vi "save_MPS_SystemRef_hdf.vi"(0 "file path":path, 1 "Device Name":tag="DAQ2", 5 "TxRx_Params":T2={"sample rate"=1000000.0, "Tx freq"=23809.52380952381, "Tx amp"=1.5, "Tx cycles\nSpectroscopy"=500.0, "Bias amp"=2.0, "Bias freq"=11.904761904761905, "Receive range"=5.0, "Bias Periods\nMagnetometry"=5.0, "Tx Freq Division Factor"=42.0, "Drive Periods per Bias"=2000.0, "TX harmonics"=[52631.57894736842, 78947.36842105263, 105263.15789473684, 131578.94736842104, 157894.73684210525, 184210.52631578947, 210526.31578947368, 236842.1052631579]} {"TX harmonics" format="%#_6p"}, 7 "Rx_f0-f8 Units":string, 11 "SRM Stats":T1={"Mean of Mags\nTF Corrected"=[0.11891545467140323, 3.2359956159889795e-06, 4.683456836791031e-06, 2.2974949759077933e-06, 7.335205151756684e-06, 2.2780944083652307e-06, 3.6882771584744806e-06, 3.943947428053956e-06, 5.677081505502577e-06], "Mean of Phase\nTF Corrected"=[1.2189052024941316, 1.3335507267391822, 1.0623290638021972, 1.2312410772168787, -2.3901914592329807, -0.9400489906160769, -0.38268681350318423, -1.5651667523229502, 2.0808572423614278], "Std of Mags\nTF Corrected"=[1.7822550794636106e-06, 1.362064067189915e-06, 1.4384290038051052e-06, 1.2224491171904712e-06, 1.5415851022050893e-06, 1.1506615886407483e-06, 1.5896649122010608e-06, 1.392010277859625e-06, 1.977168509459674e-06], "Std of Phase\nTF Corrected 4"=[0.00044396269347641464, 2.1812626503429993, 0.36980551924146593, 1.6282356086497982, 1.5207696449300456, 1.7213228694360245, 2.6615550793626337, 0.5214361017901513, 1.6763493877670135], "All Mag"=[], "All Phase"=[], "RxFFTMag_AllFreqs"=[], "RxFFTPhase_AllFreqs"=[], "Std-RxFFT_AllFreqs"=[], "Rx_PSD_AllFreqs"=[], "Std-Rx_PSD_AllFreqs"=[], "TxFFTMag_AllFreqs"=[], "TxFFTPhase_AllFreqs"=[], "Std-TxFFT_AllFreqs"=[], "freqs"=[]}, 12 "Study and Experiment Description":T4={"Study Number"=5, "Study Name"="", "UUID"="", "GUI Open Time"="", "Notes"=""}, 14 "Scanner Description":T3={"Scanner Name"="", "Hardware description"="", "Preamplifier Used"="", "Preamp Gain"=5.0, "Drive Amplifier"="", "Bias Amplifier"="", "Drive Current Monitor"="", "Bias Current Monitor"=""}, 15 "Points from home to max":i32) -> ()   [LabVIEW 2021]
uses:
  <vilib>/UPVI/lvhdf5/file.llb/LVH5F Operation.ctl
  <vilib>/Utility/miscctls.llb/LVRectTypeDef.ctl
  <vilib>/UPVI/lvhdf5/attribute.llb/LVH5A Operation.ctl
  <vilib>/UPVI/lvhdf5/group.llb/H5G_obj_t.ctl
  <vilib>/UPVI/lvhdf5/dataset.llb/LVH5D Operation.ctl
  <vilib>/UPVI/lvhdf5/identifier.llb/Not an HDF5 Refnum Constant.vi
  <vilib>/UPVI/lvhdf5/attribute.llb/Write Multiple Attributes.vi
  MPS_global_variables.vi
  <vilib>/UPVI/lvhdf5/utility.llb/Select HDF5 Dialog.vi
  <vilib>/UPVI/lvhdf5/utility.llb/Select HDF5 Dialog (Object Only).vi
  <vilib>/UPVI/lvhdf5/dataset.llb/Simple H5Dwrite (Variant).vi
  <vilib>/UPVI/lvhdf5/common.llb/To HDF5 Ref.vi
  <vilib>/UPVI/lvhdf5/dataset.llb/H5Dclose.vi
  <vilib>/UPVI/lvhdf5/attribute.llb/LVH5 Write Attributes.xnode
  <vilib>/UPVI/lvhdf5/library.llb/HDF5 Ref.ctl
  <vilib>/UPVI/lvhdf5/dataset.llb/Write Dataset with Attributes.xnode
  <vilib>/UPVI/lvhdf5/attribute.llb/Cluster to Attribute Array.xnode
  <vilib>/Utility/error.llb/Error Cluster From Error Code.vi
  <vilib>/UPVI/lvhdf5/dataset.llb/OpenCreateReplace Dataset by Element Type.vi
  <vilib>/UPVI/lvhdf5/dataspace.llb/H5Sselect_hyperslab.vi
  <vilib>/UPVI/lvhdf5/dataset.llb/H5Dwrite (Variant).vi
  <vilib>/UPVI/lvhdf5/dataset.llb/H5Dget_space.vi
  <vilib>/UPVI/lvhdf5/attribute.llb/private/LVH5AwriteWDTAttrs.vi
  <vilib>/UPVI/lvhdf5/dataspace.llb/H5Sclose.vi
  <vilib>/UPVI/lvhdf5/utility.llb/Select HDF5 Dialog (File and Object).vi
  <resource>/objmgr/daqmx.rc
  <vilib>/UPVI/lvhdf5/library.llb/HDF5 Ref.lvclass
  <vilib>/Utility/Data Type/Get Type Information.vi
  <vilib>/Utility/Data Type/NI_Data Type.lvlib
  <vilib>/Utility/Data Type/Get Cluster Information.vi
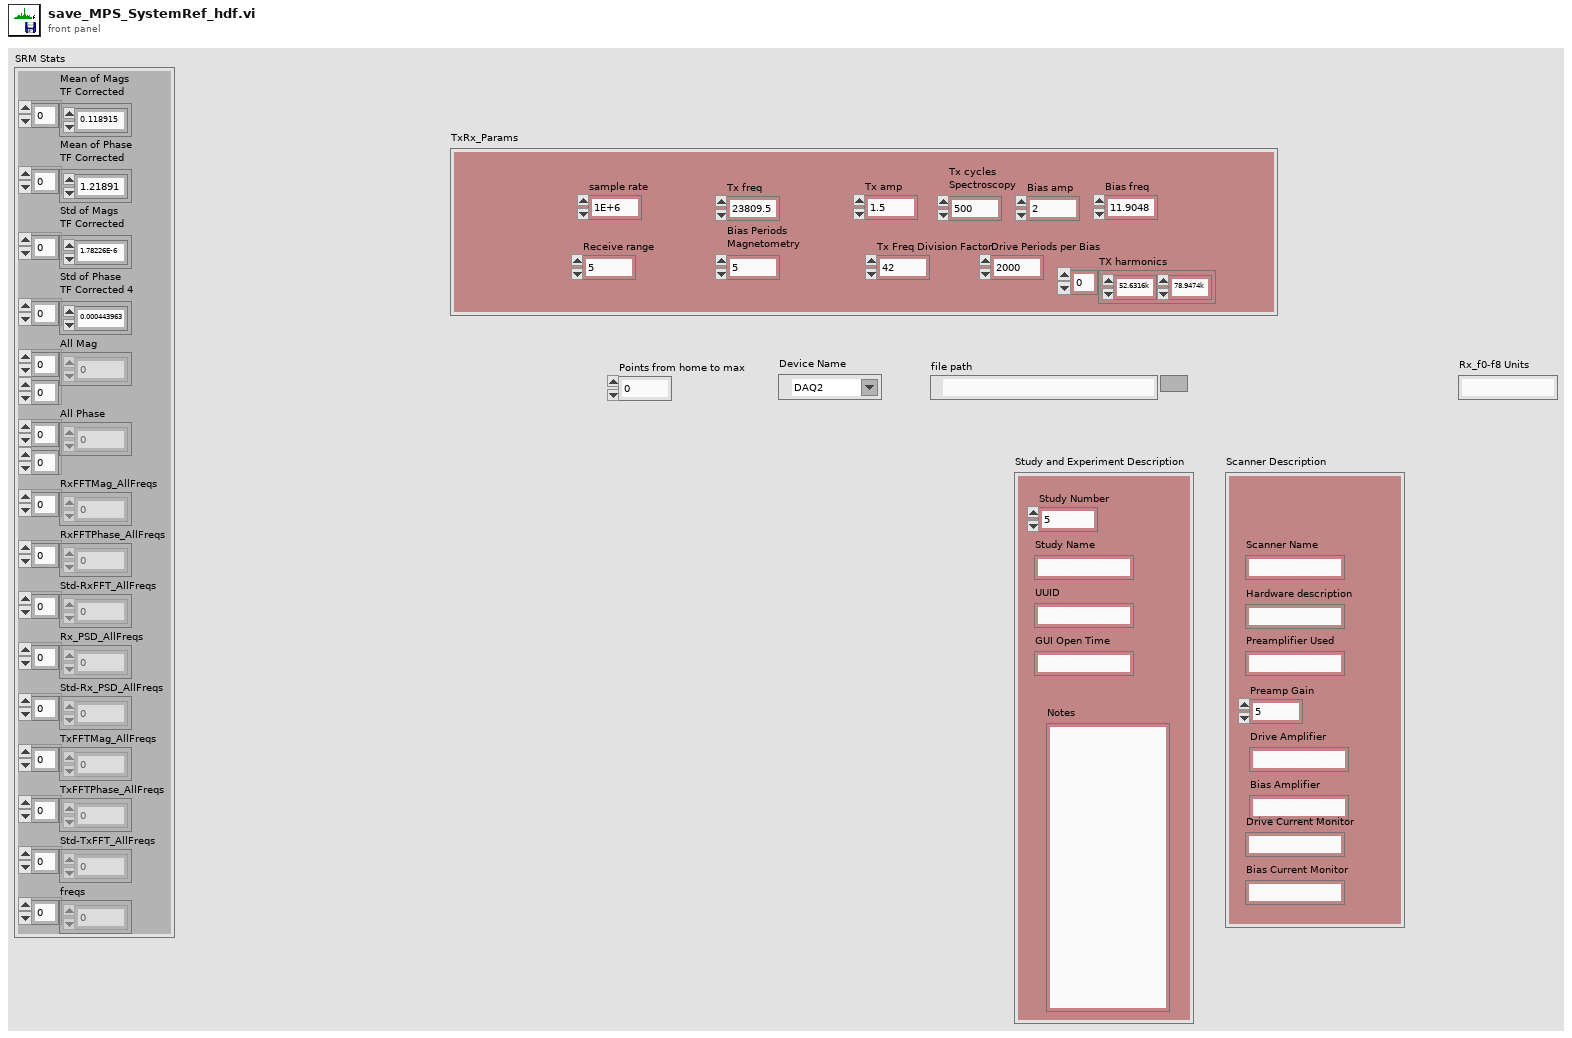
[diagram p1: front panel]
types:
  T1 = cluster{"Mean of Mags\nTF Corrected":dbl[], "Mean of Phase\nTF Corrected":dbl[], "Std of Mags\nTF Corrected":dbl[], "Std of Phase\nTF Corrected 4":dbl[], "All Mag":dbl[][], "All Phase":dbl[][], "RxFFTMag_AllFreqs":dbl[], "RxFFTPhase_AllFreqs":dbl[], "Std-RxFFT_AllFreqs":dbl[], "Rx_PSD_AllFreqs":dbl[], "Std-Rx_PSD_AllFreqs":dbl[], "TxFFTMag_AllFreqs":dbl[], "TxFFTPhase_AllFreqs":dbl[], "Std-TxFFT_AllFreqs":dbl[], "freqs":dbl[]}
  T2 = cluster{"sample rate":dbl, "Tx freq":dbl, "Tx amp":dbl, "Tx cycles\nSpectroscopy":dbl, "Bias amp":dbl, "Bias freq":dbl, "Receive range":dbl, "Bias Periods\nMagnetometry":dbl, "Tx Freq Division Factor":dbl, "Drive Periods per Bias":dbl, "TX harmonics":dbl[]}
  T3 = cluster{"Scanner Name":string, "Hardware description":string, "Preamplifier Used":string, "Preamp Gain":dbl, "Drive Amplifier":string, "Bias Amplifier":string, "Drive Current Monitor":string, "Bias Current Monitor":string}
  T4 = cluster{"Study Number":i64, "Study Name":string, "UUID":string, "GUI Open Time":string, "Notes":string}
  T5 = typedef "LVH5F Operation.ctl" = enum16{"open", "open or create", "create or replace", "create or replace (with confirmation)", "create", "open (read only)"}
  T6 = typedef "HDF5 Ref.ctl" = refnum<class "HDF5 Ref.lvclass">
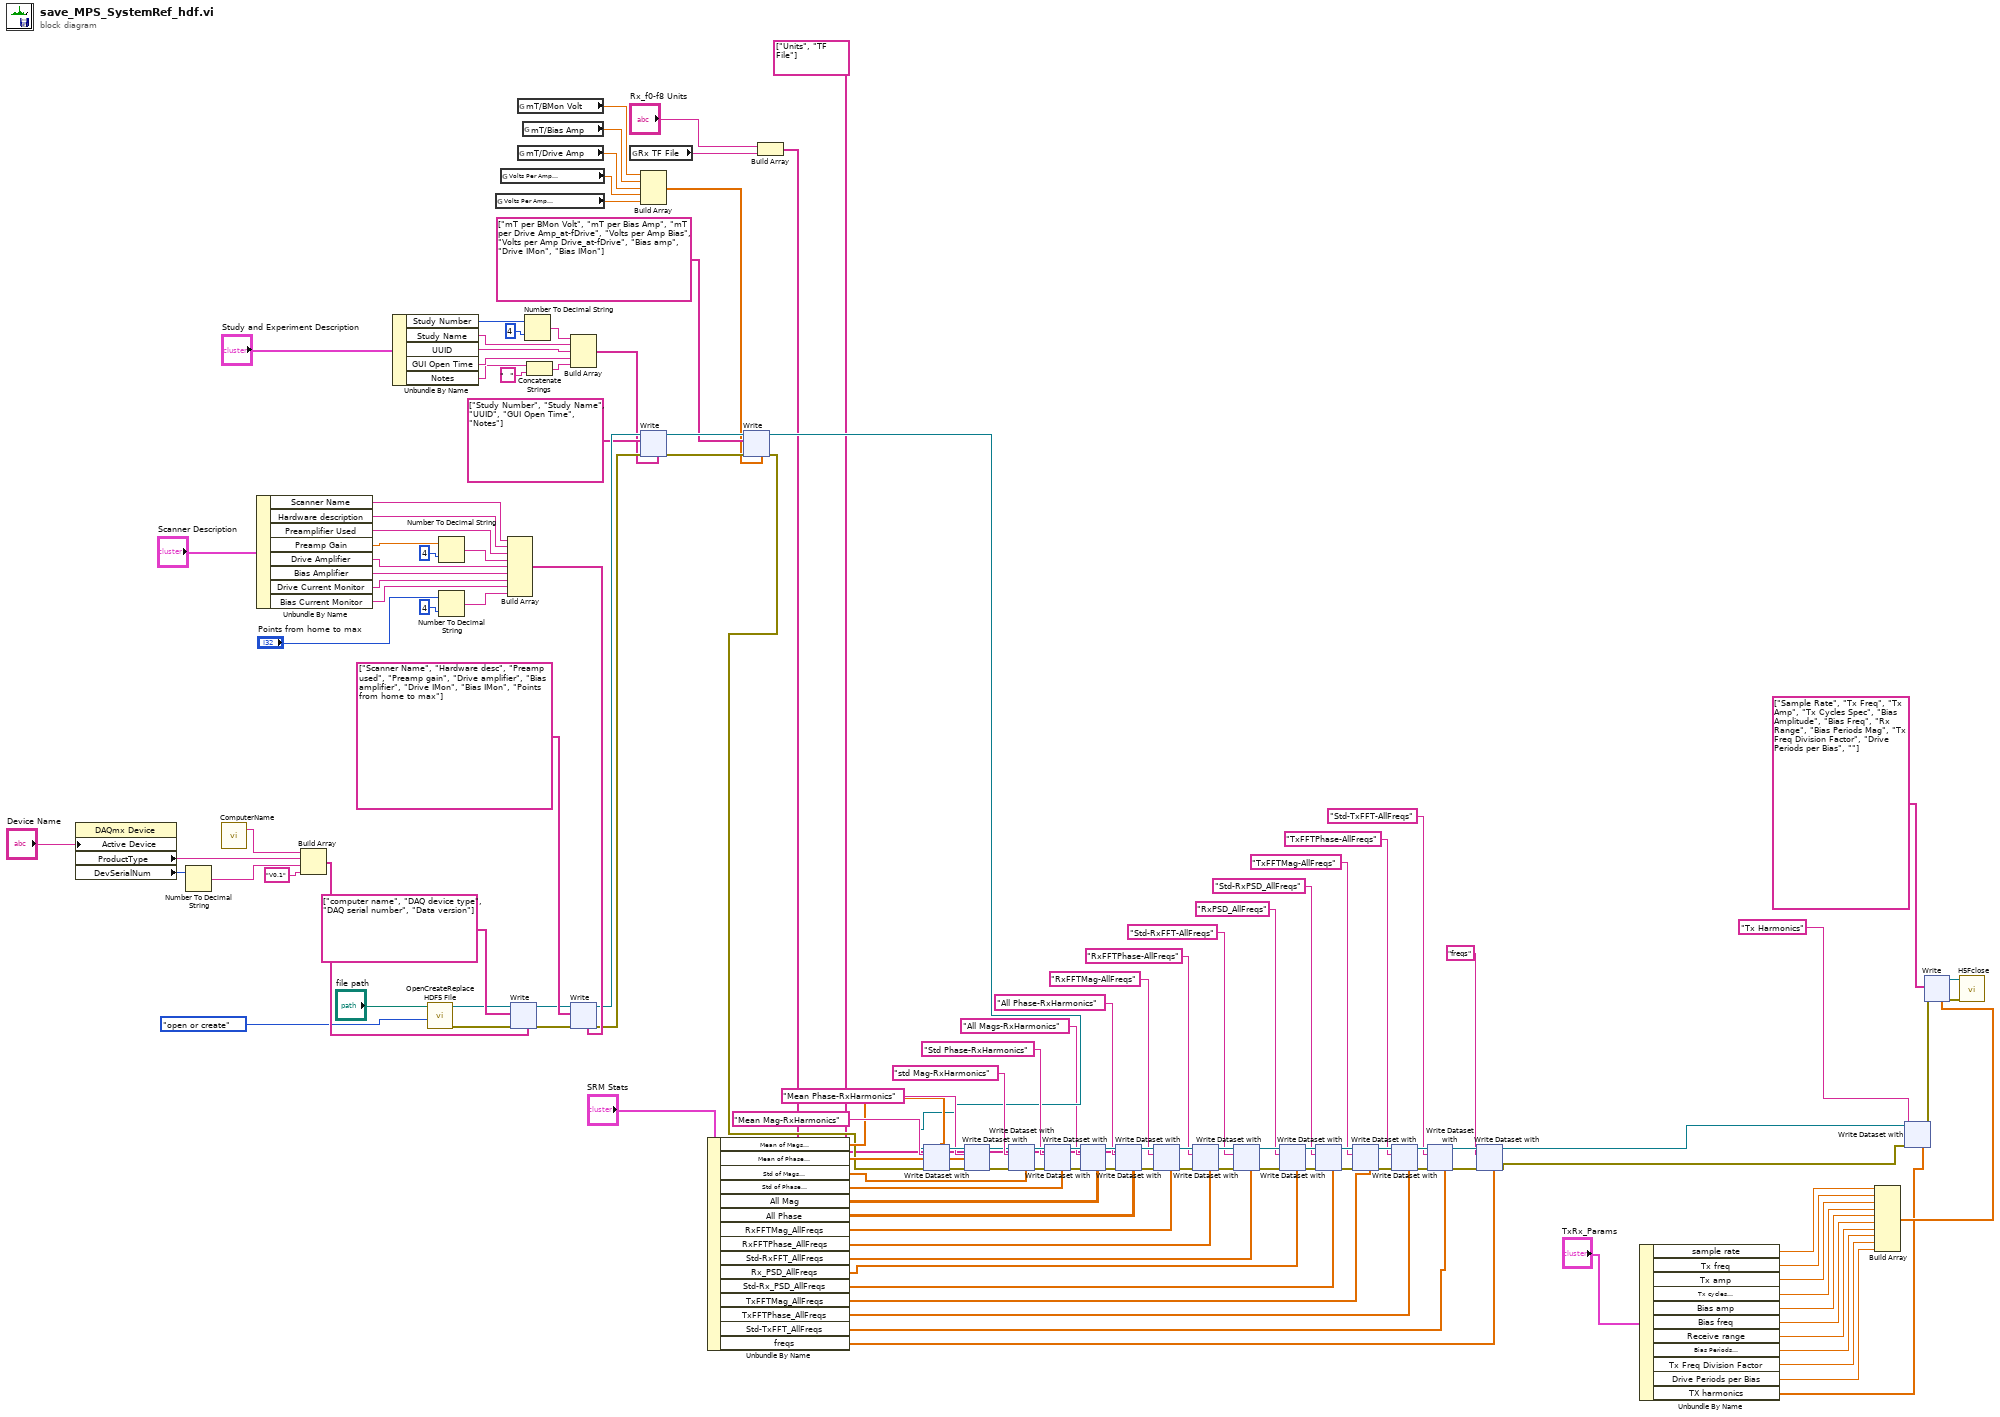
[diagram p0: block diagram]
diagram:
  w42 = string[] ["Units", "TF File"] ("Attribute Name(s)")
  n1 = property class="DAQmx Device"("Active Device"="Device Name") -> ("ProductType"=w136:string, "DevSerialNum"=w138:u32)  [unwired: 2 in, 2 out]
  n2 = Number To Decimal String(number=w138) -> (decimal integer string=w137:string)  [unwired: 1 in]
  n3 = call "ComputerName.vi"() -> ("String/Binary data"=w135:string)  [unwired: 4 in, 1 out]
  n4 = Unbundle By Name("Scanner Description") -> ("Scanner Name"=w124:string, "Hardware description"=w123:string, "Preamplifier Used"=w122:string, "Preamp Gain"=w126:dbl, "Drive Amplifier"=w120:string, "Bias Amplifier"=w119:string, "Drive Current Monitor"=w118:string, "Bias Current Monitor"=w117:string)
  n5 = Build Array(w135, w136, w137, "V0.1" ("element")) -> (w134:string[])
  n6 = Unbundle By Name("Study and Experiment Description") -> ("Study Number"=w115:i64, "Study Name"=w112:string, "UUID"=w111:string, "GUI Open Time"=w110:string, "Notes"=w83:string)
  n7 = call <vilib>:"OpenCreateReplace HDF5 File.vi"("function (open or create)"=LVH5F_Operation."open or create", "path"="file path") -> ("error out"=w129:errorcluster, "HDF5 Ref out"=w130:T6)  [unwired: 6 in]
  n8 = Number To Decimal String(number=w126, width (-)=i16 4) -> (decimal integer string=w121:string)
  n9 = Number To Decimal String(number="Points from home to max", width (-)=i16 4) -> (decimal integer string=w59:string)
  n10 = global read "MPS_global_variables.vi" "Volts Per Amp\nDrive"() -> (w64:dbl)
  n11 = global read "MPS_global_variables.vi" "Volts Per Amp\nBias"() -> (w65:dbl)
  n12 = Build Array(w124, w123, w122, w121, w120, w119, w118, w117, w59) -> (w109:string[])
  n13 = xnode "Write"("HDF5 Ref"=w130, "error in (no error)"=w129, "Name(s)"=string[] ["computer name", "DAQ device type", "DAQ serial number", "Data version"], "Value(s)"=w134) -> ("HDF5 Ref out"=w53:T6, "error out"=w52:errorcluster)  [unwired: 1 in]
  n14 = global read "MPS_global_variables.vi" "mT/BMon Volt"() -> (w68:dbl)
  n15 = global read "MPS_global_variables.vi" "mT/Drive Amp"() -> (w66:dbl)
  n16 = global read "MPS_global_variables.vi" "mT/Bias Amp"() -> (w67:dbl)
  n17 = Number To Decimal String(number=w115, width (-)=i16 4) -> (decimal integer string=w113:string)
  n18 = Concatenate Strings(w83, "  " ("string")) -> (w82:string)
  n19 = Build Array(w113, w112, w111, w110, w82) -> (w105:string[])
  n20 = xnode "Write"("HDF5 Ref"=w53, "error in (no error)"=w52, "Name(s)"=string[] ["Scanner Name", "Hardware desc", "Preamp used", "Preamp gain", "Drive amplifier", "Bias amplifier", "Drive IMon", "Bias IMon", "Points from home to max"], "Value(s)"=w109) -> ("HDF5 Ref out"=w108:T6, "error out"=w107:errorcluster)  [unwired: 1 in]
  n21 = global read "MPS_global_variables.vi" "Rx TF File"() -> (w61:string)
  n22 = Build Array(w68, w67, w66, w65, w64) -> (w62:dbl[])
  n23 = xnode "Write"("HDF5 Ref"=w108, "error in (no error)"=w107, "Name(s)"=string[] ["Study Number", "Study Name", "UUID", "GUI Open Time", "Notes"], "Value(s)"=w105) -> ("HDF5 Ref out"=w70:T6, "error out"=w69:errorcluster)  [unwired: 1 in]
  n24 = Unbundle By Name("SRM Stats") -> ("Mean of Mags\nTF Corrected"=w57:dbl[], "Mean of Phase\nTF Corrected"=w56:dbl[], "Std of Mags\nTF Corrected"=w55:dbl[], "Std of Phase\nTF Corrected 4"=w54:dbl[], "All Mag"=w41:dbl[][], "All Phase"=w40:dbl[][], "RxFFTMag_AllFreqs"=w22:dbl[], "RxFFTPhase_AllFreqs"=w21:dbl[], "Std-RxFFT_AllFreqs"=w20:dbl[], "Rx_PSD_AllFreqs"=w19:dbl[], "Std-Rx_PSD_AllFreqs"=w18:dbl[], "TxFFTMag_AllFreqs"=w17:dbl[], "TxFFTPhase_AllFreqs"=w16:dbl[], "Std-TxFFT_AllFreqs"=w15:dbl[], "freqs"=w3:dbl[])
  n25 = xnode "Write"("HDF5 Ref"=w70, "error in (no error)"=w69, "Name(s)"=string[] ["mT per BMon Volt", "mT per Bias Amp", "mT per Drive Amp_at-fDrive", "Volts per Amp Bias", "Volts per Amp Drive_at-fDrive", "Bias amp", "Drive IMon", "Bias IMon"], "Value(s)"=w62) -> ("HDF5 Ref out"=w51:T6, "error out"=w50:errorcluster)  [unwired: 1 in]
  n26 = Build Array("Rx_f0-f8 Units", w61) -> (w43:string[])
  n27 = xnode "Write Dataset with"("Dataset Path"="Mean Mag-RxHarmonics", "error in (no error)"=w50, "HDF5 Path or Ref"=w51, "Attribute Name(s)"=w42, "Attribute Value(s)"=w43, "Data"=w57) -> ("HDF5 Ref out"=w76:T6, "error out"=w74:errorcluster)  [unwired: 2 in, 1 out]
  n28 = xnode "Write Dataset with"("Dataset Path"="Mean Phase-RxHarmonics", "error in (no error)"=w74, "HDF5 Path or Ref"=w76, "Attribute Name(s)"=w42, "Attribute Value(s)"=w43, "Data"=w56) -> ("HDF5 Ref out"=w75:T6, "error out"=w73:errorcluster)  [unwired: 2 in, 1 out]
  n29 = xnode "Write Dataset with"("Dataset Path"="std Mag-RxHarmonics", "error in (no error)"=w73, "HDF5 Path or Ref"=w75, "Attribute Name(s)"=w42, "Attribute Value(s)"=w43, "Data"=w55) -> ("HDF5 Ref out"=w87:T6, "error out"=w86:errorcluster)  [unwired: 2 in, 1 out]
  n30 = xnode "Write Dataset with"("Dataset Path"="Std Phase-RxHarmonics", "error in (no error)"=w86, "HDF5 Path or Ref"=w87, "Attribute Name(s)"=w42, "Attribute Value(s)"=w43, "Data"=w54) -> ("HDF5 Ref out"=w47:T6, "error out"=w49:errorcluster)  [unwired: 2 in, 1 out]
  n31 = xnode "Write Dataset with"("Dataset Path"="All Mags-RxHarmonics", "error in (no error)"=w49, "HDF5 Path or Ref"=w47, "Data"=w41) -> ("HDF5 Ref out"=w46:T6, "error out"=w48:errorcluster)  [unwired: 4 in, 1 out]
  n32 = xnode "Write Dataset with"("Dataset Path"="All Phase-RxHarmonics", "error in (no error)"=w48, "HDF5 Path or Ref"=w46, "Attribute Name(s)"=w42, "Attribute Value(s)"=w43, "Data"=w40) -> ("HDF5 Ref out"=w33:T6, "error out"=w34:errorcluster)  [unwired: 2 in, 1 out]
  n33 = xnode "Write Dataset with"("Dataset Path"="RxFFTMag-AllFreqs", "error in (no error)"=w34, "HDF5 Path or Ref"=w33, "Data"=w22) -> ("HDF5 Ref out"=w32:T6, "error out"=w35:errorcluster)  [unwired: 4 in, 1 out]
  n34 = xnode "Write Dataset with"("Dataset Path"="RxFFTPhase-AllFreqs", "error in (no error)"=w35, "HDF5 Path or Ref"=w32, "Data"=w21) -> ("HDF5 Ref out"=w31:T6, "error out"=w36:errorcluster)  [unwired: 4 in, 1 out]
  n35 = xnode "Write Dataset with"("Dataset Path"="Std-RxFFT-AllFreqs", "error in (no error)"=w36, "HDF5 Path or Ref"=w31, "Data"=w20) -> ("HDF5 Ref out"=w30:T6, "error out"=w38:errorcluster)  [unwired: 4 in, 1 out]
  n36 = xnode "Write Dataset with"("Dataset Path"="RxPSD_AllFreqs", "error in (no error)"=w38, "HDF5 Path or Ref"=w30, "Data"=w19) -> ("HDF5 Ref out"=w29:T6, "error out"=w37:errorcluster)  [unwired: 4 in, 1 out]
  n37 = xnode "Write Dataset with"("Dataset Path"="Std-RxPSD_AllFreqs", "error in (no error)"=w37, "HDF5 Path or Ref"=w29, "Data"=w18) -> ("HDF5 Ref out"=w23:T6, "error out"=w24:errorcluster)  [unwired: 4 in, 1 out]
  n38 = xnode "Write Dataset with"("Dataset Path"="TxFFTMag-AllFreqs", "error in (no error)"=w24, "HDF5 Path or Ref"=w23, "Data"=w17) -> ("HDF5 Ref out"=w27:T6, "error out"=w25:errorcluster)  [unwired: 4 in, 1 out]
  n39 = xnode "Write Dataset with"("Dataset Path"="TxFFTPhase-AllFreqs", "error in (no error)"=w25, "HDF5 Path or Ref"=w27, "Data"=w16) -> ("HDF5 Ref out"=w28:T6, "error out"=w26:errorcluster)  [unwired: 4 in, 1 out]
  n40 = xnode "Write Dataset with"("Dataset Path"="Std-TxFFT-AllFreqs", "error in (no error)"=w26, "HDF5 Path or Ref"=w28, "Data"=w15) -> ("HDF5 Ref out"=w5:T6, "error out"=w6:errorcluster)  [unwired: 4 in, 1 out]
  n41 = xnode "Write Dataset with"("Dataset Path"="freqs", "error in (no error)"=w6, "HDF5 Path or Ref"=w5, "Data"=w3) -> ("HDF5 Ref out"=w2:T6, "error out"=w1:errorcluster)  [unwired: 4 in, 1 out]
  n42 = Unbundle By Name("TxRx_Params") -> ("sample rate"=w102:dbl, "Tx freq"=w101:dbl, "Tx amp"=w100:dbl, "Tx cycles\nSpectroscopy"=w99:dbl, "Bias amp"=w98:dbl, "Bias freq"=w97:dbl, "Receive range"=w96:dbl, "Bias Periods\nMagnetometry"=w95:dbl, "Tx Freq Division Factor"=w89:dbl, "Drive Periods per Bias"=w90:dbl, "TX harmonics"=w77:dbl[])
  n43 = Build Array(w102, w101, w100, w99, w98, w97, w96, w95, w89, w90) -> (w88:dbl[])
  n44 = xnode "Write Dataset with"("Dataset Path"="Tx Harmonics", "error in (no error)"=w1, "HDF5 Path or Ref"=w2, "Data"=w77) -> ("HDF5 Ref out"=w79:T6, "error out"=w80:errorcluster)  [unwired: 4 in, 1 out]
  n45 = xnode "Write"("HDF5 Ref"=w79, "error in (no error)"=w80, "Name(s)"=string[] ["Sample Rate", "Tx Freq", "Tx Amp", "Tx Cycles Spec", "Bias Amplitude", "Bias Freq", "Rx Range", "Bias Periods Mag", "Tx Freq Division Factor", "Drive Periods per Bias", ""], "Value(s)"=w88) -> ("HDF5 Ref out"=w104:T6, "error out"=w94:errorcluster)  [unwired: 1 in]
  n46 = call <vilib>:"H5Fclose.vi"("error in (no error)"=w94, "HDF5 Ref"=w104) -> ()  [unwired: 7 in, 1 out]
